vi "GetJointRotation.vi"(8 "error in (no error)":errorcluster, 10 "Joint":T1, 11 "JKI.Robot.SMO":refnum<class "JKI.Robot.SMO.lvclass">) -> (0 "error out":errorcluster, 1 "Rotation (Deg)":dbl, 3 "JKI.Robot.SMO out":refnum<class "JKI.Robot.SMO.lvclass">)   [LabVIEW 2014, in "JKI.Robot.SMO.lvclass"]
doc: "---------------------------------------------------------------\nJKI State Machine Objects™\nhttp://jki.net/state-machine-objects/\nCopyright (C) 2005-2015, JKI <info@jki.net>\nALL RIGHTS RESERVEDJKI State Machine Objects (SMO) 1.0.0.4\nJKI - JKI\nCopyright (c) 2015, JKI"
uses:
  JKI.Robot.SMO.lvclass
  Typedefs/JointType--Enum.ctl
  JKI.Robot.SMO.lvclass/JKI.Robot.SMO.ctl
panel:
  # "For instructions on how to use the JKI State Machine Objects, examples and video tutorials, visit:\nhttp://jki.net/state-machine-objects/\n\nJKI State Machine Objects™\nhttp://jki.net/state-machine-objects/\nCopyright (C) 2005-2015, JKI <info@jki.net>\nALL RIGHTS RESERVED"
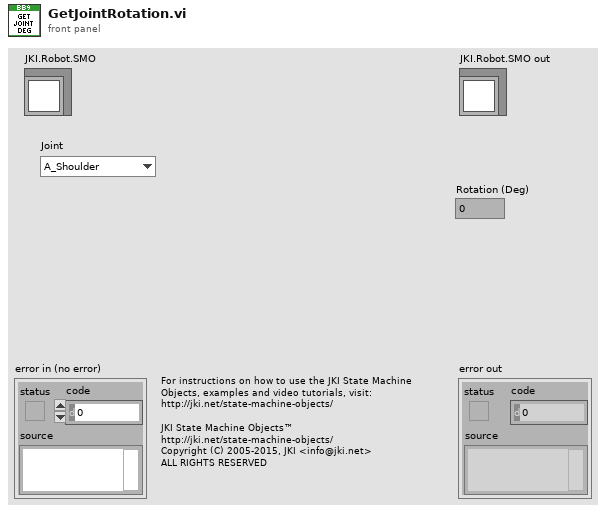
[diagram p1: front panel]
types:
  T1 = typedef "JointType--Enum.ctl" = enum16{"A_Shoulder", "B_Elbow", "C_Wrist", "D_Base"}
  T2 = typedef "JKI.Robot.SMO.lvclass/PrivateData--Ref.ctl" = refnum<data-value>
  T3 = typedef "JKI.Robot.SMO.lvclass/PrivateData--Cluster.ctl" = cluster{"Configuration":T4, "Public Events":T5, "Robot Position":T6, "Private Events":T7}
  T4 = typedef "JKI.Robot.SMO.lvclass/Configuration--Cluster.ctl" = cluster{"Suffix":string}
  T5 = typedef "JKI.Robot.SMO.lvclass/PublicEvents--Cluster.ctl" = cluster{"Data Changed":refnum<user-event>}
  T6 = typedef "RobotPosition--Cluster.ctl" = cluster{"Claw%":dbl, "JointA":dbl, "JointB":dbl, "JointC":dbl, "JointD":dbl}
  T7 = typedef "JKI.Robot.SMO.lvclass/PrivateEvents--Cluster.ctl" = cluster{"SetGrabberPosition":refnum<user-event>, "SetJointRotation":refnum<user-event>}
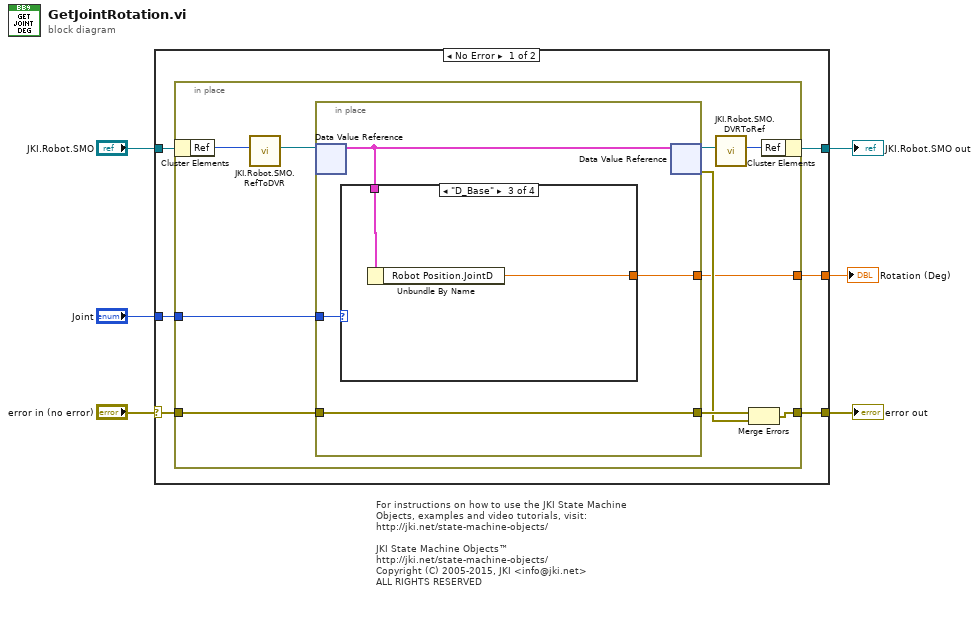
[diagram p0: block diagram]
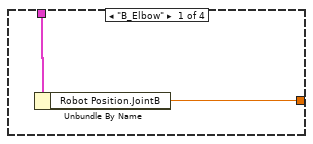
[diagram p2: hidden frame]
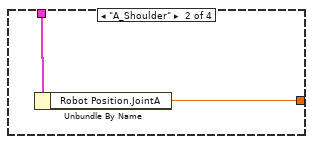
[diagram p3: hidden frame]
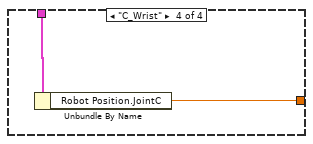
[diagram p4: hidden frame]
diagram:
  # "For instructions on how to use the JKI State Machine Objects, examples and video tutorials, visit:\nhttp://jki.net/state-machine-objects/\n\nJKI State Machine Objects™\nhttp://jki.net/state-machine-objects/\nCopyright (C) 2005-2015, JKI <info@jki.net>\nALL RIGHTS RESERVED"
  n1 = case shown="No Error" "error in (no error)" {
    selector: "error in (no error)" -> [w10 w36]
    tunnel: [w9 w36] -> w5
    tunnel: [w11 w35] -> w6
    tunnel: "JKI.Robot.SMO" -> [w12 w35]
    tunnel: "Joint" -> [w8 _]
    tunnel: [w7 _] -> w1
    frame No Error {
      n2 = in-place {
        in-place-border: w10 -> [w22]
        in-place-border: [w19] -> w9
        in-place-border: w8 -> [w14]
        in-place-border: [w13] -> w7
        n3 = in-place-cluster #1(w12) -> ("Ref"=w18:u32)
        n4 = call "JKI.Robot.SMO.RefToDVR.vi"("Ref"=w18) -> ("Ref"=w16:T2)  [unwired: 10 in]
        n5 = in-place {
          in-place-border: w22 -> [w23]
          in-place-border: [w23] -> w21
          in-place-border: w14 -> [w25]
          in-place-border: [w24] -> w13
          n6 = in-place-dvr #2(w16) -> (w26:T3)  [unwired: 1 out]
          n7 = case shown="\"D_Base\"" w25 {
            tunnel: w26 -> [w28 w30 w32 w34]
            tunnel: [w27 w29 w31 w33] -> w24
            frame "B_Elbow" {
              n8 = Unbundle By Name(w28) -> ("Robot Position.JointB"=w27:dbl)
            }
            frame "A_Shoulder" {
              n9 = Unbundle By Name(w30) -> ("Robot Position.JointA"=w29:dbl)
            }
            frame "D_Base" {
              n10 = Unbundle By Name(w32) -> ("Robot Position.JointD"=w31:dbl)
            }
            frame "C_Wrist" {
              n11 = Unbundle By Name(w34) -> ("Robot Position.JointC"=w33:dbl)
            }
          }
          n12 = in-place-dvr #2(w26) -> (w17:T2, w20:errorcluster)
        }
        n13 = call "JKI.Robot.SMO.DVRToRef.vi"("Ref"=w17) -> ("Ref"=w15:u32)  [unwired: 10 in]
        n14 = Merge Errors(w21, w20) -> (w19:errorcluster)
        n15 = in-place-cluster #1("Ref"=w15) -> (w11:refnum<class "JKI.Robot.SMO.lvclass">)
      }
    }
    frame Error {
    }
  }
  "error out" <- w5
  "JKI.Robot.SMO out" <- w6
  "Rotation (Deg)" <- w1
